vi "PLC_comm.vi"() -> ()   [LabVIEW 2017]
uses:
  <vilib>/DATA AHEAD/SP7/typedefs/PLC Type.ctl
  <vilib>/Utility/error.llb/DialogType.ctl
  <vilib>/addons/database/Connection.llb/DB Tools Open Connec (String).vi
  Global/Global 1.vi
  Global/DATA LOG.vi
  <vilib>/DATA AHEAD/SP7/functions/write/write Dint array.vi
  <vilib>/DATA AHEAD/SP7/functions/write/writeString.vi
  <vilib>/DATA AHEAD/SP7/functions/read/read Dint array.vi
  <vilib>/DATA AHEAD/SP7/functions/read/read real array.vi
  <vilib>/DATA AHEAD/SP7/functions/read/read String.vi
  <vilib>/addons/database/NI_Database_API.lvlib
  <vilib>/DATA AHEAD/SP7/SP7.lvlib
panel:
  out "IP1 7":string
  out "PLC 7":bool
  out "IP1 6":string
  out "PLC 6":bool
  out "IP1 5":string
  out "PLC 5":bool
  out "PLC 4":bool
  out "PLC 3":bool
  out "PLC 2":bool
  out "PLC 1":bool
  out "IP1 4":string
  out "IP1 3":string
  out "IP1 2":string
  out "IP1":string
  in  "stop":bool
  out "error out":errorcluster
  in  "error in (no error)":errorcluster
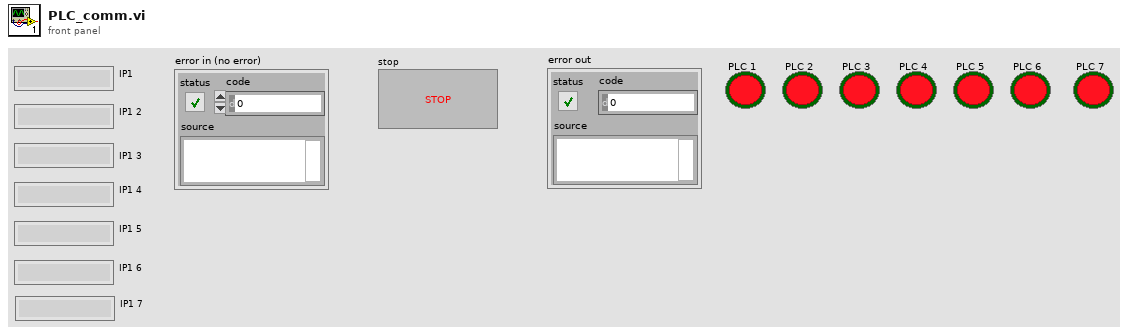
[diagram p1: front panel]
types:
  T1 = typedef "DialogType.ctl" = u16
  T2 = typedef "SP7.lvlib/PLC Type.ctl" = enum16{"S7 200", "S7 300/400", "S7 1200", "S7 1500", "LOGO!8"}
  T3 = typedef "NI_Database_API.lvlib/Conn ObjectReference.ctl" = refnum<k1>
  T4 = typedef "SP7.lvlib/S7 Connection.ctl" = cluster{"TCP Connection Ref":refnum<k5>, "IP address":string, "timeout ms":i32, "Connected?":bool, "PLC Type":T2, "Rack S7 400":u8, "Slot S7 400":u8, "PDU Size":u16, "connection semaphore":T5}
  T5 = typedef "Semaphore RefNum" = refnum<k1>
diagram:
  w2 = T1 0 items=["no dialog", "OK message", "continue or stop message", "OK message + warnings", "continue/stop + warnings"]  # type of dialog (OK msg:1)
  w4 = i32[] [0, 0, 0, 0, 0]  # I/P
  w5 = i32[] [0, 0]  # Input
  w7 = i32[] [0, 0]  # Input
  w8 = i32[] [0, 0]  # Input
  w10 = i32[] [0, 0]  # Input
  w6 = i32[] [0, 0, 0, 0, 0]  # I/P
  w9 = i32[] [0, 0, 0, 0, 0]  # I/P
  w11 = i32[] [0, 0, 0, 0, 0]  # I/P
  w12 = i32[] [0, 0, 0, 0, 0]  # I/P
  w13 = i32[] [0, 0]  # Input
  w14 = i32[] [0, 0]  # Input
  w15 = i32[] [0, 0, 0, 0, 0]  # I/P
  w16 = i32[] [0, 0, 0, 0, 0]  # I/P
  w17 = i32[] [0, 0]  # Input
  w18 = i32[] [0, 0]  # I/P
  w19 = i32[] [0, 0]  # Input
  # "OP 80"
  # "OP 70"
  # "OP 60"
  # "OP 50"
  # "OP 40"
  # "OP 30"
  # "OP 20"
  # "OP 10"
  n1 = call "path_db.vi"("error in"="error in (no error)") -> ("error out"=w174:errorcluster, "resulting string"=w179:string)  [unwired: 9 in]
  n2 = call-poly <vilib>:"DB Tools Open Connection.vi"("error in (no error)"=w174, "connection information"=w179) -> ("error out"=w178:errorcluster, "connection reference"=w177:T3)  [unwired: 6 in]
  n3 = call <vilib>:"DB Tools Select Data.vi"("error in (no error)"=w178, "columns"=string[] ["PLC_IP_1", "PLC_IP_2", "PLC_IP_3", "PLC_IP_4", "PLC_IP_5", "PLC_IP_6", "PLC_IP_7"], "table"="IP_SETTING", "connection reference"=w177) -> ("error out"=w176:errorcluster, "data"=w175:variant[][])  [unwired: 2 in, 1 out]
  n4 = call "PADMINI_varient_to_data.vi"("error in (no error)"=w176, "data"=w175) -> ("error out"=w26:errorcluster, "Array"=w170:string[][])  [unwired: 8 in]
  n5 = call "PADMINI_AUTO_CYCLE STATE.vi"("Enum"=enum16{"Read", "Write"}."Write", "error in (no error)"=w26, "Input"=w19) -> ("error out"=w156:errorcluster)  [unwired: 7 in, 1 out]
  n6 = Index Array(array=w170, index (row)=0) -> (element=w169:string[])  [unwired: 1 in]
  n7 = call "PADMINI_AUTO_BARCODE_STRING.vi"("Enum"=enum16{"Read", "Write"}."Write", "error in (no error)"=w156, "Input"=string[] ["", ""]) -> ("error out"=w153:errorcluster)  [unwired: 7 in, 1 out]
  n8 = call "PADMINI_AUTO_BARCODE_STATUS.vi"("Enum"=enum16{"Read", "Write"}."Write", "error in (no error)"=w153, "I/P"=w18) -> ("error out"=w151:errorcluster)  [unwired: 7 in, 1 out]
  n9 = call "PADMINI_AUTO_CYCLE VALUE 10.vi"("Enum"=enum16{"Read", "Write"}."Write", "error in (no error)"=w151, "Input"=dbl[] [0.0]) -> ("error out"=w145:errorcluster)  [unwired: 7 in, 1 out]
  n10 = call "PADMINI_AUTO_CYCLE STATE 20.vi"("Enum"=enum16{"Read", "Write"}."Write", "error in (no error)"=w145, "Input"=w5) -> ("error out"=w143:errorcluster)  [unwired: 7 in, 1 out]
  n11 = call "PADMINI_AUTO_CYCLE VALUE 20.vi"("Enum"=enum16{"Read", "Write"}."Write", "error in (no error)"=w143, "Input"=dbl[] [0.0, 0.0, 0.0, 0.0]) -> ("error out"=w139:errorcluster)  [unwired: 7 in, 1 out]
  n12 = call "PADMINI_AUTO_BARCODE_STRING2.vi"("Enum"=enum16{"Read", "Write"}."Write", "error in (no error)"=w139, "Input"=string[] ["", "", "", "", "", "", ""]) -> ("error out"=w137:errorcluster)  [unwired: 7 in, 1 out]
  n13 = call "PADMINI_AUTO_BARCODE_STATUS 20.vi"("Enum"=enum16{"Read", "Write"}."Write", "error in (no error)"=w137, "I/P"=w4) -> ("error out"=w131:errorcluster)  [unwired: 7 in, 1 out]
  n14 = call "PADMINI_AUTO_BARCODE_STATUS 30.vi"("Enum"=enum16{"Read", "Write"}."Write", "error in (no error)"=w131, "I/P"=w6) -> ("error out"=w128:errorcluster)  [unwired: 7 in, 1 out]
  n15 = call "PADMINI_AUTO_CYCLE STATE 30.vi"("Enum"=enum16{"Read", "Write"}."Write", "error in (no error)"=w128, "Input"=w7) -> ("error out"=w127:errorcluster)  [unwired: 7 in, 1 out]
  n16 = call "PADMINI_AUTO_CYCLE VALUE 30.vi"("Enum"=enum16{"Read", "Write"}."Write", "error in (no error)"=w127, "Input"=dbl[] [0.0, 0.0]) -> ("error out"=w124:errorcluster)  [unwired: 7 in, 1 out]
  n17 = call "PADMINI_AUTO_BARCODE_STRING 30.vi"("Enum"=enum16{"Read", "Write"}."Write", "error in (no error)"=w124, "Input"=string[] ["", "", ""]) -> ("error out"=w102:errorcluster)  [unwired: 7 in, 1 out]
  n18 = call "PADMINI_AUTO_BARCODE_STATUS 40.vi"("Enum"=enum16{"Read", "Write"}."Write", "error in (no error)"=w102, "I/P"=w9) -> ("error out"=w101:errorcluster)  [unwired: 7 in, 1 out]
  n19 = call "PADMINI_AUTO_CYCLE VALUE 40.vi"("Enum"=enum16{"Read", "Write"}."Write", "error in (no error)"=w101, "Input"=dbl[] [0.0, 0.0, 0.0, 0.0]) -> ("error out"=w100:errorcluster)  [unwired: 7 in, 1 out]
  n20 = call "PADMINI_AUTO_CYCLE STATE 40.vi"("Enum"=enum16{"Read", "Write"}."Write", "error in (no error)"=w100, "Input"=w8) -> ("error out"=w99:errorcluster)  [unwired: 7 in, 1 out]
  n21 = call "PADMINI_AUTO_BARCODE_STRING 40.vi"("Enum"=enum16{"Read", "Write"}."Write", "error in (no error)"=w99, "Input"=string[] ["", "", "", "", ""]) -> ("error out"=w81:errorcluster)  [unwired: 7 in, 1 out]
  n22 = call "PADMINI_AUTO_BARCODE_STATUS 50.vi"("Enum"=enum16{"Read", "Write"}."Write", "error in (no error)"=w81, "I/P"=w11) -> ("error out"=w83:errorcluster)  [unwired: 7 in, 1 out]
  n23 = call "PADMINI_AUTO_CYCLE STATE 50.vi"("Enum"=enum16{"Read", "Write"}."Write", "error in (no error)"=w83, "Input"=w10) -> ("error out"=w87:errorcluster)  [unwired: 7 in, 1 out]
  n24 = call "PADMINI_AUTO_CYCLE VALUE 50.vi"("Enum"=enum16{"Read", "Write"}."Write", "error in (no error)"=w87, "Input"=dbl[] [0.0, 0.0, 0.0]) -> ("error out"=w84:errorcluster)  [unwired: 7 in, 1 out]
  n25 = call "PADMINI_AUTO_BARCODE_STRING 50.vi"("Enum"=enum16{"Read", "Write"}."Write", "error in (no error)"=w84, "Input"=string[] ["", "", "", "", "", ""]) -> ("error out"=w59:errorcluster)  [unwired: 7 in, 1 out]
  n26 = call "PADMINI_AUTO_BARCODE_STATUS 60.vi"("Enum"=enum16{"Read", "Write"}."Write", "error in (no error)"=w59, "I/P"=w12) -> ("error out"=w63:errorcluster)  [unwired: 7 in, 1 out]
  n27 = call "PADMINI_AUTO_CYCLE STATE 60.vi"("Enum"=enum16{"Read", "Write"}."Write", "error in (no error)"=w63, "Input"=w13) -> ("error out"=w65:errorcluster)  [unwired: 7 in, 1 out]
  n28 = call "PADMINI_AUTO_CYCLE VALUE 60.vi"("Enum"=enum16{"Read", "Write"}."Write", "error in (no error)"=w65, "Input"=dbl[] [0.0, 0.0, 0.0, 0.0, 0.0]) -> ("error out"=w68:errorcluster)  [unwired: 7 in, 1 out]
  n29 = call "PADMINI_AUTO_BARCODE_STRING 60.vi"("Enum"=enum16{"Read", "Write"}."Write", "error in (no error)"=w68, "Input"=string[] ["", "", "", "", "", ""]) -> ("error out"=w35:errorcluster)  [unwired: 7 in, 1 out]
  n30 = call "PADMINI_AUTO_BARCODE_STATUS 70.vi"("Enum"=enum16{"Read", "Write"}."Write", "error in (no error)"=w35, "I/P"=w15) -> ("error out"=w38:errorcluster)  [unwired: 7 in, 1 out]
  n31 = call "PADMINI_AUTO_CYCLE STATE 70.vi"("Enum"=enum16{"Read", "Write"}."Read", "error in (no error)"=w38, "Input"=w14) -> ("error out"=w50:errorcluster)  [unwired: 7 in, 1 out]
  n32 = call "PADMINI_AUTO_CYCLE VALUE 70.vi"("Enum"=enum16{"Read", "Write"}."Write", "error in (no error)"=w50, "Input"=dbl[] [0.0, 0.0]) -> ("error out"=w47:errorcluster)  [unwired: 7 in, 1 out]
  n33 = call "PADMINI_AUTO_BARCODE_STRING 70.vi"("Enum"=enum16{"Read", "Write"}."Write", "error in (no error)"=w47, "Input"=string[] ["", ""]) -> ("error out"=w32:errorcluster)  [unwired: 7 in, 1 out]
  n34 = call "PADMINI_AUTO_BARCODE_STATUS 80.vi"("Enum"=enum16{"Read", "Write"}."Write", "error in (no error)"=w32, "I/P"=w16) -> ("error out"=w39:errorcluster)  [unwired: 7 in, 1 out]
  n35 = call "PADMINI_AUTO_CYCLE STATE 80.vi"("Enum"=enum16{"Read", "Write"}."Write", "error in (no error)"=w39, "Input"=w17) -> ("error out"=w43:errorcluster)  [unwired: 7 in, 1 out]
  n36 = call "PADMINI_AUTO_CYCLE VALUE 80.vi"("Enum"=enum16{"Read", "Write"}."Write", "error in (no error)"=w43, "Input"=sgl[] [0.0]) -> ("error out"=w46:errorcluster)  [unwired: 7 in, 1 out]
  n37 = call "PADMINI_AUTO_BARCODE_STRING 80.vi"("Enum"=enum16{"Read", "Write"}."Write", "error in (no error)"=w46, "Input"=string[] ["", "", ""]) -> ()  [unwired: 7 in, 2 out]
  n38 = Index Array(array=w169) -> (element #1=w118:string, element #2=w119:string, element #3=w113:string, element #4=w89:string, element #5=w71:string, element #6=w28:string, element #7=w27:string)  [unwired: 7 in]
  "IP1" <- w118
  "IP1 2" <- w119
  "IP1 3" <- w113
  "IP1 4" <- w89
  "IP1 5" <- w71
  "IP1 6" <- w28
  "IP1 7" <- w27
  n39 = call <vilib>:"connect.vi"("PLC Type"=PLC_Type."S7 1200" ("PLC Type 2"), "error in (no error)"=w26, "timeout [ms]"=1000 ("timeout [ms] 2"), "IP address"=w27) -> ("error out"=w29:errorcluster, "S7 Connection out"=w1:T4)  [unwired: 6 in]
  n40 = call <vilib>:"connect.vi"("PLC Type"=PLC_Type."S7 1200" ("PLC Type 2"), "error in (no error)"=w26, "timeout [ms]"=1000 ("timeout [ms] 2"), "IP address"=w71) -> ("error out"=w76:errorcluster, "S7 Connection out"=w75:T4)  [unwired: 6 in]
  n41 = call <vilib>:"connect.vi"("PLC Type"=PLC_Type."S7 1200" ("PLC Type 2"), "error in (no error)"=w26, "timeout [ms]"=1000 ("timeout [ms] 2"), "IP address"=w28) -> ("error out"=w56:errorcluster, "S7 Connection out"=w55:T4)  [unwired: 6 in]
  n42 = call <vilib>:"connect.vi"("PLC Type"=PLC_Type."S7 1200" ("PLC Type 2"), "error in (no error)"=w26, "timeout [ms]"=1000 ("timeout [ms] 2"), "IP address"=w89) -> ("error out"=w92:errorcluster, "S7 Connection out"=w93:T4)  [unwired: 6 in]
  n43 = call <vilib>:"connect.vi"("PLC Type"=PLC_Type."S7 1200" ("PLC Type 2"), "error in (no error)"=w26, "timeout [ms]"=1000 ("timeout [ms] 2"), "IP address"=w119) -> ("error out"=w134:errorcluster, "S7 Connection out"=w133:T4)  [unwired: 6 in]
  n44 = call <vilib>:"connect.vi"("PLC Type"=PLC_Type."S7 1200" ("PLC Type 2"), "error in (no error)"=w26, "timeout [ms]"=1000 ("timeout [ms] 2"), "IP address"=w113) -> ("error out"=w115:errorcluster, "S7 Connection out"=w114:T4)  [unwired: 6 in]
  n45 = call <vilib>:"connect.vi"("PLC Type"=PLC_Type."S7 1200" ("PLC Type 2"), "error in (no error)"=w26, "timeout [ms]"=1000, "IP address"=w118) -> ("error out"=w160:errorcluster, "S7 Connection out"=w159:T4)  [unwired: 6 in]
  n46 = while {
    shift-right: [w182] -> w23
    shift-left: w1 -> [w192]
    shift-right: [w190] -> w24
    shift-left: w29 -> [w191]
    tunnel: w27 -> [w181]
    stop <- w184 stop-if-true
    # "OP 90 - 100 - 110"
    n47 = flat-sequence {
      tunnel: [w268] -> w188
      tunnel: [w269] -> w183
      tunnel: w191 -> [w307]
      tunnel: w192 -> [w306]
      tunnel: w181 -> [w288]
      tunnel: [w288] -> w180
      tunnel: [w375] -> w190
      tunnel: [w374] -> w182
      tunnel: w188 -> [w377]
      tunnel: w183 -> [w376]
      tunnel: w180 -> [w373]
      frame #0 {
        w209 = u16 75 ("Data Block #")
        w234 = u16 72 ("Data Block #")
        w260 = u16 70 ("Data Block #")
        w218 = u16 71 ("Data Block #")
        w248 = u16 69 ("Data Block #")
        # "OP100 OK\nOP 100 NG"
        # "AUTO WRITE"
        n48 = global read "DATA LOG.vi" "OP 90 Outputs"() -> (w305:bool)
        n49 = case shown="True" w305 {
          tunnel: w306 -> [w358 w371]
          tunnel: [w359 w360] -> w265
          tunnel: [w358 w361] -> w266
          tunnel: w307 -> [w359 w368]
          frame False {
          }
          frame True {
            w372 = u16 70  # Data Block #
            n50 = call "PADMINI_AUTO_BARCODE_STATUS 90.vi"("Enum"=enum16{"Read", "Write"}."Read", "error in (no error)"=w368) -> ("error out"=w367:errorcluster, "O/P"=w369:i32[])  [unwired: 8 in]
            n51 = global write "DATA LOG.vi" "OP 90 Outputs"(FALSE) -> ()
            n52 = call-poly <vilib>:"write DB.vi"("DINT input array"=w369, "error in (no error)"=w367, "Data Block #"=w372, "S7 Connection in"=w371) -> ("error out"=w363:errorcluster, "S7 Connection out"=w362:T4)  [unwired: 4 in, 2 out]
            n53 = call-poly <vilib>:"write DB.vi"("DINT input array"=i32[] [0] ("Data Byte"), "error in (no error)"=w363, "Data Block #"=u16 69, "S7 Connection in"=w362) -> ("error out"=w360:errorcluster, "S7 Connection out"=w361:T4)  [unwired: 4 in, 2 out]
          }
        }
        n54 = global read "DATA LOG.vi" "OP 90 reset"() -> (w264:bool)
        n55 = case shown="True" w264 {
          tunnel: w265 -> [w333 w342]
          tunnel: [w333 w341] -> w253
          tunnel: w266 -> [w334 w340]
          tunnel: [w334 w339] -> w254
          frame False {
          }
          frame True {
            n56 = global write "DATA LOG.vi" "OP 90 reset"(FALSE) -> ()
            n57 = call-poly <vilib>:"write DB.vi"("Item offset [byte]"=u16 4 ("Data Block #"), "DINT input array"=i32[] [0], "error in (no error)"=w342, "Data Block #"=u16 69, "S7 Connection in"=w340) -> ("error out"=w341:errorcluster, "S7 Connection out"=w339:T4)  [unwired: 3 in, 2 out]
          }
        }
        n58 = global read "DATA LOG.vi" "Auto Cycle On"() -> (w200:bool)
        n59 = Boolean To (0,1)(Boolean=w200) -> (0, 1=w199:i16)
        n60 = Build Array(w199) -> (w198:i16[])
        n61 = global read "Global 1.vi" "Filtered BARCODE selected"() -> (w263:string[])
        n62 = call-poly <vilib>:"write DB.vi"("Item offset [byte]"=u32 20, "DINT input array"=w198, "error in (no error)"=w253, "Data Block #"=w260, "S7 Connection in"=w254) -> ("error out"=w258:errorcluster, "S7 Connection out"=w257:T4)  [unwired: 3 in, 2 out]
        n63 = call-poly <vilib>:"write DB.vi"("Item offset [byte]"=u32 24, "Input STRINGS"=w263, "error in (no error)"=w258, "String length reserved in DB (default=254)"=u16 15, "Data Block #"=w260, "S7 Connection in"=w257) -> ("error out"=w255:errorcluster, "S7 Connection out"=w256:T4)  [unwired: 2 in, 2 out]
        n64 = call-poly <vilib>:"read DB.vi"("error in (no error)"=w255, "items #"=u16 2 ("Items # [byte]"), "Data Block #"=w248, "S7 Connection in"=w256) -> ("error out"=w303:errorcluster, "DINT result array"=w301:i32[], "S7 Connection out"=w298:T4)  [unwired: 5 in]
        n65 = call "PADMINI_AUTO_CYCLE STATE 90.vi"("Enum"=enum16{"Read", "Write"}."Write", "error in (no error)"=w303, "Input"=w301) -> ("error out"=w299:errorcluster)  [unwired: 7 in, 1 out]
        n66 = call-poly <vilib>:"read DB.vi"("Item offset [byte]"=u32 8, "error in (no error)"=w299, "items #"=u16 2 ("Items # [byte]"), "Data Block #"=w248, "S7 Connection in"=w298) -> ("error out"=w291:errorcluster, "REAL result array"=w289:sgl[], "S7 Connection out"=w297:T4)  [unwired: 4 in]
        n67 = call "PADMINI_AUTO_CYCLE VALUE 90.vi"("Enum"=enum16{"Read", "Write"}."Write", "error in (no error)"=w291, "Input"=w289) -> ("error out"=w290:errorcluster)  [unwired: 7 in, 1 out]
        n68 = call-poly <vilib>:"read DB.vi"("Item offset [byte]"=u32 16, "String length reserved in DB (default=254)"=u16 50, "error in (no error)"=w290, "items #"=u16 1 ("Items # [byte]"), "Data Block #"=w248, "S7 Connection in"=w297) -> ("error out"=w252:errorcluster, "STRING result Array"=w243:string[], "S7 Connection out"=w251:T4)  [unwired: 2 in, 1 out]
        n69 = call-poly <vilib>:"read DB.vi"("Item offset [byte]"=u32 68, "String length reserved in DB (default=254)"=u16 10, "error in (no error)"=w252, "items #"=u16 3 ("Items # [byte]"), "Data Block #"=w248, "S7 Connection in"=w251) -> ("error out"=w250:errorcluster, "STRING result Array"=w242:string[], "S7 Connection out"=w249:T4)  [unwired: 2 in, 1 out]
        n70 = Build Array (concatenate)(w243, w242) -> (w241:string[])
        n71 = call "PADMINI_AUTO_BARCODE_STRING 90.vi"("Enum"=enum16{"Read", "Write"}."Write", "error in (no error)"=w250, "Input"=w241) -> ("error out"=w270:errorcluster)  [unwired: 7 in, 1 out]
        n72 = global read "DATA LOG.vi" "OP 100 Outputs"() -> (w271:bool)
        n73 = case shown="True" w271 {
          tunnel: w249 -> [w343 w356]
          tunnel: [w344 w347] -> w239
          tunnel: [w343 w348] -> w240
          tunnel: w270 -> [w344 w353]
          frame False {
          }
          frame True {
            w357 = u16 72  # Data Block #
            n74 = call "PADMINI_AUTO_BARCODE_STATUS 100.vi"("Enum"=enum16{"Read", "Write"}."Read", "error in (no error)"=w353) -> ("error out"=w352:errorcluster, "O/P"=w354:i32[])  [unwired: 8 in]
            n75 = global write "DATA LOG.vi" "OP 100 Outputs"(FALSE) -> ()
            n76 = call-poly <vilib>:"write DB.vi"("DINT input array"=w354, "error in (no error)"=w352, "Data Block #"=w357, "S7 Connection in"=w356) -> ("error out"=w346:errorcluster, "S7 Connection out"=w345:T4)  [unwired: 4 in, 2 out]
            n77 = call-poly <vilib>:"write DB.vi"("DINT input array"=i32[] [0] ("Data Byte"), "error in (no error)"=w346, "Data Block #"=u16 71, "S7 Connection in"=w345) -> ("error out"=w347:errorcluster, "S7 Connection out"=w348:T4)  [unwired: 4 in, 2 out]
          }
        }
        n78 = global read "DATA LOG.vi" "OP 100 reset"() -> (w238:bool)
        n79 = case shown="True" w238 {
          tunnel: w239 -> [w323 w332]
          tunnel: [w323 w331] -> w230
          tunnel: w240 -> [w324 w330]
          tunnel: [w324 w329] -> w229
          frame False {
          }
          frame True {
            n80 = global write "DATA LOG.vi" "OP 100 reset"(FALSE) -> ()
            n81 = call-poly <vilib>:"write DB.vi"("Item offset [byte]"=u16 4 ("Data Block #"), "DINT input array"=i32[] [0], "error in (no error)"=w332, "Data Block #"=u16 71, "S7 Connection in"=w330) -> ("error out"=w331:errorcluster, "S7 Connection out"=w329:T4)  [unwired: 3 in, 2 out]
          }
        }
        n82 = global read "DATA LOG.vi" "Auto Cycle On"() -> (w197:bool)
        n83 = Boolean To (0,1)(Boolean=w197) -> (0, 1=w196:i16)
        n84 = Build Array(w196) -> (w195:i16[])
        n85 = global read "Global 1.vi" "Filtered BARCODE selected"() -> (w231:string[])
        n86 = call-poly <vilib>:"write DB.vi"("Item offset [byte]"=u32 20, "DINT input array"=w195, "error in (no error)"=w230, "Data Block #"=w234, "S7 Connection in"=w229) -> ("error out"=w236:errorcluster, "S7 Connection out"=w237:T4)  [unwired: 3 in, 2 out]
        n87 = call-poly <vilib>:"write DB.vi"("Item offset [byte]"=u32 24, "Input STRINGS"=w231, "error in (no error)"=w236, "String length reserved in DB (default=254)"=u16 15, "Data Block #"=w234, "S7 Connection in"=w237) -> ("error out"=w227:errorcluster, "S7 Connection out"=w228:T4)  [unwired: 2 in, 2 out]
        n88 = call-poly <vilib>:"read DB.vi"("error in (no error)"=w227, "items #"=u16 2 ("Items # [byte]"), "Data Block #"=w218, "S7 Connection in"=w228) -> ("error out"=w273:errorcluster, "DINT result array"=w275:i32[], "S7 Connection out"=w278:T4)  [unwired: 5 in]
        n89 = call "PADMINI_AUTO_CYCLE STATE 100.vi"("Enum"=enum16{"Read", "Write"}."Write", "error in (no error)"=w273, "Input"=w275) -> ("error out"=w277:errorcluster)  [unwired: 7 in, 1 out]
        n90 = call-poly <vilib>:"read DB.vi"("Item offset [byte]"=u32 8, "error in (no error)"=w277, "items #"=u16 11 ("Items # [byte]"), "Data Block #"=w218, "S7 Connection in"=w278) -> ("error out"=w285:errorcluster, "REAL result array"=w287:sgl[], "S7 Connection out"=w279:T4)  [unwired: 4 in]
        n91 = call "PADMINI_AUTO_CYCLE VALUE 100.vi"("Enum"=enum16{"Read", "Write"}."Write", "error in (no error)"=w285, "Input"=w287) -> ("error out"=w286:errorcluster)  [unwired: 7 in, 1 out]
        n92 = call-poly <vilib>:"read DB.vi"("Item offset [byte]"=u32 52, "String length reserved in DB (default=254)"=u16 50, "error in (no error)"=w286, "items #"=u16 1 ("Items # [byte]"), "Data Block #"=w218, "S7 Connection in"=w279) -> ("error out"=w224:errorcluster, "STRING result Array"=w221:string[], "S7 Connection out"=w223:T4)  [unwired: 2 in, 1 out]
        n93 = call-poly <vilib>:"read DB.vi"("Item offset [byte]"=u32 104, "String length reserved in DB (default=254)"=u16 10, "error in (no error)"=w224, "items #"=u16 2 ("Items # [byte]"), "Data Block #"=w218, "S7 Connection in"=w223) -> ("error out"=w225:errorcluster, "STRING result Array"=w219:string[], "S7 Connection out"=w222:T4)  [unwired: 2 in, 1 out]
        n94 = Build Array (concatenate)(w221, w219) -> (w220:string[])
        n95 = call "PADMINI_AUTO_BARCODE_STRING 100.vi"("Enum"=enum16{"Read", "Write"}."Write", "error in (no error)"=w225, "Input"=w220) -> ("error out"=w267:errorcluster)  [unwired: 7 in, 1 out]
        n96 = global read "DATA LOG.vi" "OP 110 Outputs"() -> (w215:bool)
        n97 = case shown="True" w215 {
          tunnel: [w308 w313] -> w201
          tunnel: [w309 w314] -> w202
          tunnel: w267 -> [w308 w318]
          tunnel: w222 -> [w309 w317]
          frame False {
          }
          frame True {
            w310 = i32[] [0]  # DINT input array
            w311 = u16 75  # Data Block #
            n98 = call "PADMINI_AUTO_BARCODE_STATUS 110.vi"("Enum"=enum16{"Read", "Write"}."Read", "error in (no error)"=w318) -> ("error out"=w320:errorcluster, "O/P"=w321:i32[])  [unwired: 8 in]
            n99 = call-poly <vilib>:"write DB.vi"("Item offset [byte]"=u32 4, "DINT input array"=w321, "error in (no error)"=w320, "Data Block #"=w311, "S7 Connection in"=w317) -> ("error out"=w312:errorcluster, "S7 Connection out"=w315:T4)  [unwired: 3 in, 2 out]
            n100 = global write "DATA LOG.vi" "OP 110 Outputs"(FALSE) -> ()
            n101 = call-poly <vilib>:"write DB.vi"("DINT input array"=w310, "error in (no error)"=w312, "Data Block #"=w311, "S7 Connection in"=w315) -> ("error out"=w313:errorcluster, "S7 Connection out"=w314:T4)  [unwired: 4 in, 2 out]
          }
        }
        n102 = call-poly <vilib>:"read DB.vi"("error in (no error)"=w201, "items #"=u16 1 ("Items # [byte]"), "Data Block #"=w209, "S7 Connection in"=w202) -> ("error out"=w213:errorcluster, "DINT result array"=w211:i32[], "S7 Connection out"=w210:T4)  [unwired: 5 in]
        n103 = call "PADMINI_AUTO_CYCLE STATE 110.vi"("Enum"=enum16{"Read", "Write"}."Write", "error in (no error)"=w213, "Input"=w211) -> ("error out"=w203:errorcluster)  [unwired: 7 in, 1 out]
        n104 = call-poly <vilib>:"read DB.vi"("Item offset [byte]"=u32 12, "String length reserved in DB (default=254)"=u16 50, "error in (no error)"=w203, "items #"=u16 1 ("Items # [byte]"), "Data Block #"=w209, "S7 Connection in"=w210) -> ("error out"=w205:errorcluster, "STRING result Array"=w206:string[], "S7 Connection out"=w268:T4)  [unwired: 2 in, 1 out]
        n105 = call "PADMINI_AUTO_BARCODE_STRING 110.vi"("Enum"=enum16{"Read", "Write"}."Write", "error in (no error)"=w205, "Input"=w206) -> ("error out"=w269:errorcluster)  [unwired: 7 in, 1 out]
      }
      frame #1 {
        # "RECONNECT"
        n106 = case shown="Error" w376 {
          selector: w376 -> [w381 w389]
          tunnel: [w380 w386] -> w374
          tunnel: [w381 w387] -> w375
          tunnel: w377 -> [w380 w383]
          tunnel: w373 -> [_ w382]
          frame No Error {
          }
          frame Error {
            n107 = call <vilib>:"Clear Errors.vi"("error in (no error)"=w389) -> ("error out"=w390:errorcluster)  [unwired: 5 in, 1 out]
            n108 = call <vilib>:"disconnect.vi"("error in (no error)"=w390, "S7 Connection in"=w383) -> ("error out"=w388:errorcluster)  [unwired: 8 in, 1 out]
            n109 = call <vilib>:"Clear Errors.vi"("error in (no error)"=w388) -> ("error out"=w385:errorcluster)  [unwired: 5 in, 1 out]
            n110 = call <vilib>:"connect.vi"("PLC Type"=PLC_Type."S7 1200" ("PLC Type 2"), "error in (no error)"=w385, "IP address"=w382) -> ("error out"=w387:errorcluster, "S7 Connection out"=w386:T4)  [unwired: 7 in]
          }
        }
        n111 = Unbundle By Name(w376) -> ("status"=w379:bool)
        n112 = Not(x=w379) -> (.not. x?=w378:bool)
        "PLC 7" <- w378
        n113 = global write "Global 1.vi" "PLC 7"(w378) -> ()
      }
    }
    n114 = call "PADMINI_STOP_ALL.vi"("Enum"=enum16{"Read", "Write"}."Read") -> ("Boolean 2"=w186:bool)  [unwired: 9 in, 1 out]
    n115 = local read "stop"() -> (w185:bool)
    n116 = Or(x=w185, y=w186) -> (x .or. y?=w184:bool)
    n117 = Wait (ms)(milliseconds to wait=u32 50) -> ()  [unwired: 1 out]
  }
  n118 = while {
    shift-right: [w393] -> w121
    shift-left: w133 -> [w403]
    shift-right: [w401] -> w120
    shift-left: w134 -> [w402]
    tunnel: w119 -> [w392]
    stop <- w395 stop-if-true
    # "OP 30"
    n119 = flat-sequence {
      tunnel: [w406] -> w399
      tunnel: [w408] -> w394
      tunnel: w402 -> [w410]
      tunnel: w403 -> [w409]
      tunnel: w392 -> [w407]
      tunnel: [w407] -> w391
      tunnel: [w413] -> w401
      tunnel: [w412] -> w393
      tunnel: w399 -> [w415]
      tunnel: w394 -> [w414]
      tunnel: w391 -> [w411]
      frame #0 {
        # "AUTO WRITE"
        n120 = call "PLC_OP30_Write.vi"("error in (no error)"=w410, "S7 Connection in"=w409) -> ("error out"=w404:errorcluster, "S7 Connection out"=w405:T4)  [unwired: 8 in]
        n121 = call "PLC_OP30_Read.vi"("error in (no error)"=w404, "S7 Connection in"=w405) -> ("error out"=w408:errorcluster, "S7 Connection out 2"=w406:T4)  [unwired: 8 in]
      }
      frame #1 {
        # "RECONNECT"
        n122 = case shown="Error" w414 {
          selector: w414 -> [w419 w427]
          tunnel: [w418 w424] -> w412
          tunnel: [w419 w425] -> w413
          tunnel: w415 -> [w418 w421]
          tunnel: w411 -> [_ w420]
          frame No Error {
          }
          frame Error {
            n123 = call <vilib>:"Clear Errors.vi"("error in (no error)"=w427) -> ("error out"=w428:errorcluster)  [unwired: 5 in, 1 out]
            n124 = call <vilib>:"disconnect.vi"("error in (no error)"=w428, "S7 Connection in"=w421) -> ("error out"=w426:errorcluster)  [unwired: 8 in, 1 out]
            n125 = call <vilib>:"Clear Errors.vi"("error in (no error)"=w426) -> ("error out"=w423:errorcluster)  [unwired: 5 in, 1 out]
            n126 = call <vilib>:"connect.vi"("PLC Type"=PLC_Type."S7 1200" ("PLC Type 2"), "error in (no error)"=w423, "IP address"=w420) -> ("error out"=w425:errorcluster, "S7 Connection out"=w424:T4)  [unwired: 7 in]
          }
        }
        n127 = Unbundle By Name(w414) -> ("status"=w417:bool)
        n128 = Not(x=w417) -> (.not. x?=w416:bool)
        "PLC 2" <- w416
        n129 = global write "Global 1.vi" "PLC 2"(w416) -> ()
      }
    }
    n130 = call "PADMINI_STOP_ALL.vi"("Enum"=enum16{"Read", "Write"}."Read") -> ("Boolean 2"=w397:bool)  [unwired: 9 in, 1 out]
    n131 = Wait (ms)(milliseconds to wait=u32 50) -> ()  [unwired: 1 out]
    n132 = local read "stop"() -> (w396:bool)
    n133 = Or(x=w396, y=w397) -> (x .or. y?=w395:bool)
  }
  n134 = while {
    shift-right: [w431] -> w148
    shift-left: w159 -> [w441]
    shift-right: [w439] -> w163
    shift-left: w160 -> [w440]
    tunnel: w118 -> [w429]
    stop <- w434 stop-if-true
    # "OP 10 AND 20"
    n135 = flat-sequence {
      tunnel: [w444] -> w433
      tunnel: [w450] -> w432
      tunnel: w440 -> [w451]
      tunnel: w441 -> [w452]
      tunnel: [w449] -> w430
      tunnel: w429 -> [w449]
      tunnel: [w456] -> w439
      tunnel: [w455] -> w431
      tunnel: w433 -> [w457]
      tunnel: w432 -> [w453]
      tunnel: w430 -> [w454]
      frame #0 {
        # "NEW CHANGES"
        n136 = call "PLC_OP10_Write.vi"("error in (no error)"=w451, "S7 Connection in"=w452) -> ("error out"=w447:errorcluster, "S7 Connection out"=w448:T4)  [unwired: 8 in]
        n137 = call "PLC_OP10_Read.vi"("error in (no error)"=w447, "S7 Connection in"=w448) -> ("error out"=w446:errorcluster, "S7 Connection out"=w445:T4)  [unwired: 8 in]
        n138 = call "PLC_OP20_Write.vi"("error in (no error)"=w446, "S7 Connection in"=w445) -> ("error out"=w442:errorcluster, "S7 Connection out"=w443:T4)  [unwired: 8 in]
        n139 = call "PLC_OP20_Read.vi"("error in (no error)"=w442, "S7 Connection in"=w443) -> ("error out"=w450:errorcluster, "S7 Connection out 2"=w444:T4)  [unwired: 8 in]
      }
      frame #1 {
        # "RECONNECT"
        n140 = Unbundle By Name(w453) -> ("status"=w459:bool)
        n141 = case shown="Error" w453 {
          selector: w453 -> [w461 w470]
          tunnel: [w460 w467] -> w455
          tunnel: [w461 w468] -> w456
          tunnel: w457 -> [w460 w464]
          tunnel: w454 -> [_ w463]
          frame No Error {
          }
          frame Error {
            w462 = 1000  # timeout [ms]
            n142 = call <vilib>:"Clear Errors.vi"("error in (no error)"=w470) -> ("error out"=w471:errorcluster)  [unwired: 5 in, 1 out]
            n143 = call <vilib>:"disconnect.vi"("error in (no error)"=w471, "S7 Connection in"=w464) -> ("error out"=w469:errorcluster)  [unwired: 8 in, 1 out]
            n144 = call <vilib>:"Clear Errors.vi"("error in (no error)"=w469) -> ("error out"=w466:errorcluster)  [unwired: 5 in, 1 out]
            n145 = call <vilib>:"connect.vi"("PLC Type"=PLC_Type."S7 1200" ("PLC Type 2"), "error in (no error)"=w466, "timeout [ms]"=w462, "IP address"=w463) -> ("error out"=w468:errorcluster, "S7 Connection out"=w467:T4)  [unwired: 6 in]
          }
        }
        n146 = Not(x=w459) -> (.not. x?=w458:bool)
        "PLC 1" <- w458
        n147 = global write "Global 1.vi" "PLC 1"(w458) -> ()
      }
    }
    n148 = call "PADMINI_STOP_ALL.vi"("Enum"=enum16{"Read", "Write"}."Read") -> ("Boolean 2"=w436:bool)  [unwired: 9 in, 1 out]
    n149 = Or(x="stop", y=w436) -> (x .or. y?=w434:bool)
    n150 = Wait (ms)(milliseconds to wait=u32 50) -> ()  [unwired: 1 out]
  }
  n151 = while {
    shift-right: [w474] -> w96
    shift-left: w93 -> [w484]
    shift-right: [w482] -> w95
    shift-left: w92 -> [w483]
    tunnel: w89 -> [w473]
    stop <- w476 stop-if-true
    # "OP 50"
    n152 = flat-sequence {
      tunnel: [w505] -> w480
      tunnel: [w515] -> w475
      tunnel: w483 -> [w534]
      tunnel: w484 -> [w533]
      tunnel: w473 -> [w514]
      tunnel: [w514] -> w472
      tunnel: [w562] -> w482
      tunnel: [w561] -> w474
      tunnel: w480 -> [w564]
      tunnel: w475 -> [w563]
      tunnel: w472 -> [w560]
      frame #0 {
        w496 = u16 57 ("Data Block #")
        w504 = u16 56 ("Data Block #")
        # "AUTO WRITE"
        n153 = global read "DATA LOG.vi" "OP 50 Outputs"() -> (w532:bool)
        n154 = case shown="True" w532 {
          tunnel: w533 -> [w545 w558]
          tunnel: [w546 w547] -> w513
          tunnel: [w545 w550] -> w512
          tunnel: w534 -> [w546 w555]
          frame False {
          }
          frame True {
            w559 = u16 57  # Data Block #
            n155 = call "PADMINI_AUTO_BARCODE_STATUS 50.vi"("Enum"=enum16{"Read", "Write"}."Read", "error in (no error)"=w555) -> ("error out"=w554:errorcluster, "O/P"=w556:i32[])  [unwired: 8 in]
            n156 = global write "DATA LOG.vi" "OP 50 Outputs"(FALSE) -> ()
            n157 = call-poly <vilib>:"write DB.vi"("DINT input array"=w556, "error in (no error)"=w554, "Data Block #"=w559, "S7 Connection in"=w558) -> ("error out"=w548:errorcluster, "S7 Connection out"=w549:T4)  [unwired: 4 in, 2 out]
            n158 = call-poly <vilib>:"write DB.vi"("DINT input array"=i32[] [0] ("Data Byte"), "error in (no error)"=w548, "Data Block #"=u16 56, "S7 Connection in"=w549) -> ("error out"=w547:errorcluster, "S7 Connection out"=w550:T4)  [unwired: 4 in, 2 out]
          }
        }
        n159 = global read "DATA LOG.vi" "OP 50 reset"() -> (w511:bool)
        n160 = global read "DATA LOG.vi" "Auto Cycle On"() -> (w487:bool)
        n161 = case shown="True" w511 {
          tunnel: w513 -> [w535 w544]
          tunnel: [w535 w543] -> w489
          tunnel: w512 -> [w536 w542]
          tunnel: [w536 w541] -> w492
          frame False {
          }
          frame True {
            n162 = global write "DATA LOG.vi" "OP 50 reset"(FALSE) -> ()
            n163 = call-poly <vilib>:"write DB.vi"("Item offset [byte]"=u16 4 ("Data Block #"), "DINT input array"=i32[] [0], "error in (no error)"=w544, "Data Block #"=u16 56, "S7 Connection in"=w542) -> ("error out"=w543:errorcluster, "S7 Connection out"=w541:T4)  [unwired: 3 in, 2 out]
          }
        }
        n164 = Boolean To (0,1)(Boolean=w487) -> (0, 1=w486:i16)
        n165 = Build Array(w486) -> (w485:i16[])
        n166 = global read "Global 1.vi" "Filtered BARCODE selected"() -> (w493:string[])
        n167 = call-poly <vilib>:"write DB.vi"("Item offset [byte]"=u32 20, "DINT input array"=w485, "error in (no error)"=w489, "Data Block #"=w496, "S7 Connection in"=w492) -> ("error out"=w498:errorcluster, "S7 Connection out"=w499:T4)  [unwired: 3 in, 2 out]
        n168 = call-poly <vilib>:"write DB.vi"("Item offset [byte]"=u32 24, "Input STRINGS"=w493, "error in (no error)"=w498, "String length reserved in DB (default=254)"=u16 15, "Data Block #"=w496, "S7 Connection in"=w499) -> ("error out"=w490:errorcluster, "S7 Connection out"=w491:T4)  [unwired: 2 in, 2 out]
        n169 = call-poly <vilib>:"read DB.vi"("error in (no error)"=w490, "items #"=u16 2 ("Items # [byte]"), "Data Block #"=w504, "S7 Connection in"=w491) -> ("error out"=w530:errorcluster, "DINT result array"=w528:i32[], "S7 Connection out"=w525:T4)  [unwired: 5 in]
        n170 = call "PADMINI_AUTO_CYCLE STATE 50.vi"("Enum"=enum16{"Read", "Write"}."Write", "error in (no error)"=w530, "Input"=w528) -> ("error out"=w526:errorcluster)  [unwired: 7 in, 1 out]
        n171 = call-poly <vilib>:"read DB.vi"("Item offset [byte]"=u32 8, "error in (no error)"=w526, "items #"=u16 3 ("Items # [byte]"), "Data Block #"=w504, "S7 Connection in"=w525) -> ("error out"=w518:errorcluster, "REAL result array"=w516:sgl[], "S7 Connection out"=w524:T4)  [unwired: 4 in]
        n172 = call "PADMINI_AUTO_CYCLE VALUE 50.vi"("Enum"=enum16{"Read", "Write"}."Write", "error in (no error)"=w518, "Input"=w516) -> ("error out"=w517:errorcluster)  [unwired: 7 in, 1 out]
        n173 = call-poly <vilib>:"read DB.vi"("Item offset [byte]"=u32 20, "String length reserved in DB (default=254)"=u16 50, "error in (no error)"=w517, "items #"=u16 1 ("Items # [byte]"), "Data Block #"=w504, "S7 Connection in"=w524) -> ("error out"=w507:errorcluster, "STRING result Array"=w503:string[], "S7 Connection out"=w506:T4)  [unwired: 2 in, 1 out]
        n174 = call-poly <vilib>:"read DB.vi"("Item offset [byte]"=u32 72, "String length reserved in DB (default=254)"=u16 10, "error in (no error)"=w507, "items #"=u16 5 ("Items # [byte]"), "Data Block #"=w504, "S7 Connection in"=w506) -> ("error out"=w508:errorcluster, "STRING result Array"=w502:string[], "S7 Connection out"=w505:T4)  [unwired: 2 in, 1 out]
        n175 = Build Array (concatenate)(w503, w502) -> (w501:string[])
        n176 = call "PADMINI_AUTO_BARCODE_STRING 50.vi"("Enum"=enum16{"Read", "Write"}."Write", "error in (no error)"=w508, "Input"=w501) -> ("error out"=w515:errorcluster)  [unwired: 7 in, 1 out]
      }
      frame #1 {
        # "RECONNECT"
        n177 = case shown="Error" w563 {
          selector: w563 -> [w568 w576]
          tunnel: [w567 w573] -> w561
          tunnel: [w568 w574] -> w562
          tunnel: w564 -> [w567 w570]
          tunnel: w560 -> [_ w569]
          frame No Error {
          }
          frame Error {
            n178 = call <vilib>:"Clear Errors.vi"("error in (no error)"=w576) -> ("error out"=w577:errorcluster)  [unwired: 5 in, 1 out]
            n179 = call <vilib>:"disconnect.vi"("error in (no error)"=w577, "S7 Connection in"=w570) -> ("error out"=w575:errorcluster)  [unwired: 8 in, 1 out]
            n180 = call <vilib>:"Clear Errors.vi"("error in (no error)"=w575) -> ("error out"=w572:errorcluster)  [unwired: 5 in, 1 out]
            n181 = call <vilib>:"connect.vi"("PLC Type"=PLC_Type."S7 1200" ("PLC Type 2"), "error in (no error)"=w572, "IP address"=w569) -> ("error out"=w574:errorcluster, "S7 Connection out"=w573:T4)  [unwired: 7 in]
          }
        }
        n182 = Unbundle By Name(w563) -> ("status"=w566:bool)
        n183 = Not(x=w566) -> (.not. x?=w565:bool)
        "PLC 4" <- w565
        n184 = global write "Global 1.vi" "PLC 4"(w565) -> ()
      }
    }
    n185 = call "PADMINI_STOP_ALL.vi"("Enum"=enum16{"Read", "Write"}."Read") -> ("Boolean 2"=w478:bool)  [unwired: 9 in, 1 out]
    n186 = local read "stop"() -> (w477:bool)
    n187 = Or(x=w477, y=w478) -> (x .or. y?=w476:bool)
    n188 = Wait (ms)(milliseconds to wait=u32 50) -> ()  [unwired: 1 out]
  }
  n189 = while {
    shift-right: [w580] -> w52
    shift-left: w55 -> [w590]
    shift-right: [w588] -> w53
    shift-left: w56 -> [w589]
    tunnel: w28 -> [w579]
    stop <- w582 stop-if-true
    # "OP 70 - 80"
    n190 = flat-sequence {
      tunnel: [w601] -> w586
      tunnel: [w649] -> w581
      tunnel: w589 -> [w687]
      tunnel: w590 -> [w686]
      tunnel: w579 -> [w668]
      tunnel: [w668] -> w578
      tunnel: [w740] -> w588
      tunnel: [w739] -> w580
      tunnel: w586 -> [w742]
      tunnel: w581 -> [w741]
      tunnel: w578 -> [w738]
      frame #0 {
        w617 = u16 83 ("Data Block #")
        w642 = u16 81 ("Data Block #")
        w600 = u16 82 ("Data Block #")
        w623 = u16 80 ("Data Block #")
        # "AUTO WRITE"
        n191 = global read "DATA LOG.vi" "OP 70 Outputs"() -> (w685:bool)
        n192 = case shown="True" w685 {
          tunnel: w686 -> [w723 w736]
          tunnel: [w724 w727] -> w647
          tunnel: [w723 w728] -> w646
          tunnel: w687 -> [w724 w733]
          frame False {
          }
          frame True {
            w737 = u16 81  # Data Block #
            n193 = call "PADMINI_AUTO_BARCODE_STATUS 70.vi"("Enum"=enum16{"Read", "Write"}."Read", "error in (no error)"=w733) -> ("error out"=w732:errorcluster, "O/P"=w734:i32[])  [unwired: 8 in]
            n194 = global write "DATA LOG.vi" "OP 70 Outputs"(FALSE) -> ()
            n195 = call-poly <vilib>:"write DB.vi"("DINT input array"=w734, "error in (no error)"=w732, "Data Block #"=w737, "S7 Connection in"=w736) -> ("error out"=w725:errorcluster, "S7 Connection out"=w726:T4)  [unwired: 4 in, 2 out]
            n196 = call-poly <vilib>:"write DB.vi"("DINT input array"=i32[] [0] ("Data Byte"), "error in (no error)"=w725, "Data Block #"=u16 80, "S7 Connection in"=w726) -> ("error out"=w727:errorcluster, "S7 Connection out"=w728:T4)  [unwired: 4 in, 2 out]
          }
        }
        n197 = global read "DATA LOG.vi" "OP 70 reset"() -> (w648:bool)
        n198 = global read "DATA LOG.vi" "Auto Cycle On"() -> (w593:bool)
        n199 = case shown="True" w648 {
          tunnel: w647 -> [w698 w707]
          tunnel: [w698 w706] -> w637
          tunnel: w646 -> [w699 w705]
          tunnel: [w699 w704] -> w638
          frame False {
          }
          frame True {
            n200 = global write "DATA LOG.vi" "OP 70 reset"(FALSE) -> ()
            n201 = call-poly <vilib>:"write DB.vi"("Item offset [byte]"=u16 4 ("Data Block #"), "DINT input array"=i32[] [0], "error in (no error)"=w707, "Data Block #"=u16 80, "S7 Connection in"=w705) -> ("error out"=w706:errorcluster, "S7 Connection out"=w704:T4)  [unwired: 3 in, 2 out]
          }
        }
        n202 = Boolean To (0,1)(Boolean=w593) -> (0, 1=w592:i16)
        n203 = Build Array(w592) -> (w591:i16[])
        n204 = global read "Global 1.vi" "Filtered BARCODE selected"() -> (w639:string[])
        n205 = call-poly <vilib>:"write DB.vi"("Item offset [byte]"=u32 20, "DINT input array"=w591, "error in (no error)"=w637, "Data Block #"=w642, "S7 Connection in"=w638) -> ("error out"=w644:errorcluster, "S7 Connection out"=w645:T4)  [unwired: 3 in, 2 out]
        n206 = call-poly <vilib>:"write DB.vi"("Item offset [byte]"=u32 24, "Input STRINGS"=w639, "error in (no error)"=w644, "String length reserved in DB (default=254)"=u16 15, "Data Block #"=w642, "S7 Connection in"=w645) -> ("error out"=w635:errorcluster, "S7 Connection out"=w636:T4)  [unwired: 2 in, 2 out]
        n207 = call-poly <vilib>:"read DB.vi"("error in (no error)"=w635, "items #"=u16 2 ("Items # [byte]"), "Data Block #"=w623, "S7 Connection in"=w636) -> ("error out"=w683:errorcluster, "DINT result array"=w681:i32[], "S7 Connection out"=w678:T4)  [unwired: 5 in]
        n208 = call "PADMINI_AUTO_CYCLE STATE 70.vi"("Enum"=enum16{"Read", "Write"}."Write", "error in (no error)"=w683, "Input"=w681) -> ("error out"=w679:errorcluster)  [unwired: 7 in, 1 out]
        n209 = call-poly <vilib>:"read DB.vi"("Item offset [byte]"=u32 8, "error in (no error)"=w679, "items #"=u16 2 ("Items # [byte]"), "Data Block #"=w623, "S7 Connection in"=w678) -> ("error out"=w671:errorcluster, "REAL result array"=w669:sgl[], "S7 Connection out"=w677:T4)  [unwired: 4 in]
        n210 = call "PADMINI_AUTO_CYCLE VALUE 70.vi"("Enum"=enum16{"Read", "Write"}."Write", "error in (no error)"=w671, "Input"=w669) -> ("error out"=w670:errorcluster)  [unwired: 7 in, 1 out]
        n211 = call-poly <vilib>:"read DB.vi"("Item offset [byte]"=u32 16, "String length reserved in DB (default=254)"=u16 50, "error in (no error)"=w670, "items #"=u16 1 ("Items # [byte]"), "Data Block #"=w623, "S7 Connection in"=w677) -> ("error out"=w628:errorcluster, "STRING result Array"=w627:string[], "S7 Connection out"=w629:T4)  [unwired: 2 in, 1 out]
        n212 = call-poly <vilib>:"read DB.vi"("Item offset [byte]"=u32 68, "String length reserved in DB (default=254)"=u16 10, "error in (no error)"=w628, "items #"=u16 1 ("Items # [byte]"), "Data Block #"=w623, "S7 Connection in"=w629) -> ("error out"=w630:errorcluster, "STRING result Array"=w631:string[], "S7 Connection out"=w624:T4)  [unwired: 2 in, 1 out]
        n213 = Build Array (concatenate)(w627, w631) -> (w625:string[])
        n214 = call "PADMINI_AUTO_BARCODE_STRING 70.vi"("Enum"=enum16{"Read", "Write"}."Write", "error in (no error)"=w630, "Input"=w625) -> ("error out"=w650:errorcluster)  [unwired: 7 in, 1 out]
        n215 = global read "DATA LOG.vi" "OP 80 Outputs"() -> (w651:bool)
        n216 = case shown="True" w651 {
          tunnel: [w709 w712] -> w622
          tunnel: [w708 w713] -> w598
          tunnel: w650 -> [w709 w719]
          tunnel: w624 -> [w708 w716]
          frame False {
          }
          frame True {
            w722 = u16 83  # Data Block #
            n217 = call "PADMINI_AUTO_BARCODE_STATUS 80.vi"("Enum"=enum16{"Read", "Write"}."Read", "error in (no error)"=w719) -> ("error out"=w718:errorcluster, "O/P"=w720:i32[])  [unwired: 8 in]
            n218 = global write "DATA LOG.vi" "OP 80 Outputs"(FALSE) -> ()
            n219 = call-poly <vilib>:"write DB.vi"("DINT input array"=w720, "error in (no error)"=w718, "Data Block #"=w722, "S7 Connection in"=w716) -> ("error out"=w710:errorcluster, "S7 Connection out"=w711:T4)  [unwired: 4 in, 2 out]
            n220 = call-poly <vilib>:"write DB.vi"("DINT input array"=i32[] [0] ("Data Byte"), "error in (no error)"=w710, "Data Block #"=u16 82, "S7 Connection in"=w711) -> ("error out"=w712:errorcluster, "S7 Connection out"=w713:T4)  [unwired: 4 in, 2 out]
          }
        }
        n221 = global read "DATA LOG.vi" "OP 80 reset"() -> (w621:bool)
        n222 = global read "DATA LOG.vi" "Auto Cycle On"() -> (w596:bool)
        n223 = case shown="True" w621 {
          tunnel: w622 -> [w689 w697]
          tunnel: [w689 w692] -> _
          tunnel: [w689 w692] -> w611
          tunnel: w598 -> [w688 w691]
          tunnel: [w688 w690] -> w597
          frame False {
          }
          frame True {
            n224 = global write "DATA LOG.vi" "OP 80 reset"(FALSE) -> ()
            n225 = call-poly <vilib>:"write DB.vi"("Item offset [byte]"=u16 4 ("Data Block #"), "DINT input array"=i32[] [0], "error in (no error)"=w697, "Data Block #"=u16 82, "S7 Connection in"=w691) -> ("error out"=w692:errorcluster, "S7 Connection out"=w690:T4)  [unwired: 3 in, 2 out]
          }
        }
        n226 = Boolean To (0,1)(Boolean=w596) -> (0, 1=w595:i16)
        n227 = Build Array(w595) -> (w594:i16[])
        n228 = global read "Global 1.vi" "Filtered BARCODE selected"() -> (w614:string[])
        n229 = call-poly <vilib>:"write DB.vi"("Item offset [byte]"=u32 20, "DINT input array"=w594, "error in (no error)"=w611, "Data Block #"=w617, "S7 Connection in"=w597) -> ("error out"=w619:errorcluster, "S7 Connection out"=w620:T4)  [unwired: 3 in, 2 out]
        n230 = call-poly <vilib>:"write DB.vi"("Item offset [byte]"=u32 24, "Input STRINGS"=w614, "error in (no error)"=w619, "String length reserved in DB (default=254)"=u16 15, "Data Block #"=w617, "S7 Connection in"=w620) -> ("error out"=w612:errorcluster, "S7 Connection out"=w613:T4)  [unwired: 2 in, 2 out]
        n231 = call-poly <vilib>:"read DB.vi"("error in (no error)"=w612, "items #"=u16 2 ("Items # [byte]"), "Data Block #"=w600, "S7 Connection in"=w613) -> ("error out"=w653:errorcluster, "DINT result array"=w655:i32[], "S7 Connection out"=w658:T4)  [unwired: 5 in]
        n232 = call "PADMINI_AUTO_CYCLE STATE 80.vi"("Enum"=enum16{"Read", "Write"}."Write", "error in (no error)"=w653, "Input"=w655) -> ("error out"=w657:errorcluster)  [unwired: 7 in, 1 out]
        n233 = call-poly <vilib>:"read DB.vi"("Item offset [byte]"=u32 8, "error in (no error)"=w657, "items #"=u16 1 ("Items # [byte]"), "Data Block #"=w600, "S7 Connection in"=w658) -> ("error out"=w665:errorcluster, "REAL result array"=w667:sgl[], "S7 Connection out"=w659:T4)  [unwired: 4 in]
        n234 = call "PADMINI_AUTO_CYCLE VALUE 80.vi"("Enum"=enum16{"Read", "Write"}."Write", "error in (no error)"=w665, "Input"=w667) -> ("error out"=w666:errorcluster)  [unwired: 7 in, 1 out]
        n235 = call-poly <vilib>:"read DB.vi"("Item offset [byte]"=u32 12, "String length reserved in DB (default=254)"=u16 50, "error in (no error)"=w666, "items #"=u16 1 ("Items # [byte]"), "Data Block #"=w600, "S7 Connection in"=w659) -> ("error out"=w606:errorcluster, "STRING result Array"=w604:string[], "S7 Connection out"=w602:T4)  [unwired: 2 in, 1 out]
        n236 = call-poly <vilib>:"read DB.vi"("Item offset [byte]"=u32 64, "String length reserved in DB (default=254)"=u16 10, "error in (no error)"=w606, "items #"=u16 2 ("Items # [byte]"), "Data Block #"=w600, "S7 Connection in"=w602) -> ("error out"=w605:errorcluster, "STRING result Array"=w610:string[], "S7 Connection out"=w601:T4)  [unwired: 2 in, 1 out]
        n237 = Build Array (concatenate)(w604, w610) -> (w603:string[])
        n238 = call "PADMINI_AUTO_BARCODE_STRING 80.vi"("Enum"=enum16{"Read", "Write"}."Write", "error in (no error)"=w605, "Input"=w603) -> ("error out"=w649:errorcluster)  [unwired: 7 in, 1 out]
      }
      frame #1 {
        # "RECONNECT"
        n239 = case shown="Error" w741 {
          selector: w741 -> [w746 w754]
          tunnel: [w745 w751] -> w739
          tunnel: [w746 w752] -> w740
          tunnel: w742 -> [w745 w748]
          tunnel: w738 -> [_ w747]
          frame No Error {
          }
          frame Error {
            n240 = call <vilib>:"Clear Errors.vi"("error in (no error)"=w754) -> ("error out"=w755:errorcluster)  [unwired: 5 in, 1 out]
            n241 = call <vilib>:"disconnect.vi"("error in (no error)"=w755, "S7 Connection in"=w748) -> ("error out"=w753:errorcluster)  [unwired: 8 in, 1 out]
            n242 = call <vilib>:"Clear Errors.vi"("error in (no error)"=w753) -> ("error out"=w750:errorcluster)  [unwired: 5 in, 1 out]
            n243 = call <vilib>:"connect.vi"("PLC Type"=PLC_Type."S7 1200" ("PLC Type 2"), "error in (no error)"=w750, "IP address"=w747) -> ("error out"=w752:errorcluster, "S7 Connection out"=w751:T4)  [unwired: 7 in]
          }
        }
        n244 = Unbundle By Name(w741) -> ("status"=w744:bool)
        n245 = Not(x=w744) -> (.not. x?=w743:bool)
        "PLC 6" <- w743
        n246 = global write "Global 1.vi" "PLC 6"(w743) -> ()
      }
    }
    n247 = call "PADMINI_STOP_ALL.vi"("Enum"=enum16{"Read", "Write"}."Read") -> ("Boolean 2"=w584:bool)  [unwired: 9 in, 1 out]
    n248 = local read "stop"() -> (w583:bool)
    n249 = Or(x=w583, y=w584) -> (x .or. y?=w582:bool)
    n250 = Wait (ms)(milliseconds to wait=u32 50) -> ()  [unwired: 1 out]
  }
  n251 = while {
    shift-right: [w758] -> w72
    shift-left: w75 -> [w768]
    shift-right: [w766] -> w73
    shift-left: w76 -> [w767]
    tunnel: w71 -> [w757]
    stop <- w760 stop-if-true
    # "OP 60"
    n252 = flat-sequence {
      tunnel: [w777] -> w764
      tunnel: [w799] -> w759
      tunnel: w767 -> [w818]
      tunnel: w768 -> [w817]
      tunnel: w757 -> [w798]
      tunnel: [w798] -> w756
      tunnel: [w846] -> w766
      tunnel: [w845] -> w758
      tunnel: w764 -> [w848]
      tunnel: w759 -> [w847]
      tunnel: w756 -> [w844]
      frame #0 {
        w794 = u16 44 ("Data Block #")
        w774 = u16 43 ("Data Block #")
        # "AUTO WRITE"
        n253 = global read "DATA LOG.vi" "OP 60 Outputs"() -> (w816:bool)
        n254 = case shown="True" w816 {
          tunnel: w817 -> [w829 w842]
          tunnel: [w830 w831] -> w786
          tunnel: [w829 w834] -> w785
          tunnel: w818 -> [w830 w839]
          frame False {
          }
          frame True {
            w843 = u16 44  # Data Block #
            n255 = call "PADMINI_AUTO_BARCODE_STATUS 60.vi"("Enum"=enum16{"Read", "Write"}."Read", "error in (no error)"=w839) -> ("error out"=w838:errorcluster, "O/P"=w840:i32[])  [unwired: 8 in]
            n256 = global write "DATA LOG.vi" "OP 60 Outputs"(FALSE) -> ()
            n257 = call-poly <vilib>:"write DB.vi"("DINT input array"=w840, "error in (no error)"=w838, "Data Block #"=w843, "S7 Connection in"=w842) -> ("error out"=w832:errorcluster, "S7 Connection out"=w833:T4)  [unwired: 4 in, 2 out]
            n258 = call-poly <vilib>:"write DB.vi"("DINT input array"=i32[] [0] ("Data Byte"), "error in (no error)"=w832, "Data Block #"=u16 43, "S7 Connection in"=w833) -> ("error out"=w831:errorcluster, "S7 Connection out"=w834:T4)  [unwired: 4 in, 2 out]
          }
        }
        n259 = global read "DATA LOG.vi" "OP 60 reset"() -> (w784:bool)
        n260 = global read "DATA LOG.vi" "Auto Cycle On"() -> (w771:bool)
        n261 = case shown="True" w784 {
          tunnel: w786 -> [w819 w828]
          tunnel: [w819 w827] -> w787
          tunnel: w785 -> [w820 w826]
          tunnel: [w820 w825] -> w788
          frame False {
          }
          frame True {
            n262 = global write "DATA LOG.vi" "OP 60 reset"(FALSE) -> ()
            n263 = call-poly <vilib>:"write DB.vi"("Item offset [byte]"=u16 4 ("Data Block #"), "DINT input array"=i32[] [0], "error in (no error)"=w828, "Data Block #"=u16 43, "S7 Connection in"=w826) -> ("error out"=w827:errorcluster, "S7 Connection out"=w825:T4)  [unwired: 3 in, 2 out]
          }
        }
        n264 = Boolean To (0,1)(Boolean=w771) -> (0, 1=w770:i16)
        n265 = Build Array(w770) -> (w769:i16[])
        n266 = global read "Global 1.vi" "Filtered BARCODE selected"() -> (w797:string[])
        n267 = call-poly <vilib>:"write DB.vi"("Item offset [byte]"=u32 20, "DINT input array"=w769, "error in (no error)"=w787, "Data Block #"=w794, "S7 Connection in"=w788) -> ("error out"=w792:errorcluster, "S7 Connection out"=w791:T4)  [unwired: 3 in, 2 out]
        n268 = call-poly <vilib>:"write DB.vi"("Item offset [byte]"=u32 24, "Input STRINGS"=w797, "error in (no error)"=w792, "String length reserved in DB (default=254)"=u16 15, "Data Block #"=w794, "S7 Connection in"=w791) -> ("error out"=w789:errorcluster, "S7 Connection out"=w790:T4)  [unwired: 2 in, 2 out]
        n269 = call-poly <vilib>:"read DB.vi"("error in (no error)"=w789, "items #"=u16 2 ("Items # [byte]"), "Data Block #"=w774, "S7 Connection in"=w790) -> ("error out"=w814:errorcluster, "DINT result array"=w812:i32[], "S7 Connection out"=w809:T4)  [unwired: 5 in]
        n270 = call "PADMINI_AUTO_CYCLE STATE 60.vi"("Enum"=enum16{"Read", "Write"}."Write", "error in (no error)"=w814, "Input"=w812) -> ("error out"=w810:errorcluster)  [unwired: 7 in, 1 out]
        n271 = call-poly <vilib>:"read DB.vi"("Item offset [byte]"=u32 8, "error in (no error)"=w810, "items #"=u16 6 ("Items # [byte]"), "Data Block #"=w774, "S7 Connection in"=w809) -> ("error out"=w802:errorcluster, "REAL result array"=w800:sgl[], "S7 Connection out"=w808:T4)  [unwired: 4 in]
        n272 = call "PADMINI_AUTO_CYCLE VALUE 60.vi"("Enum"=enum16{"Read", "Write"}."Write", "error in (no error)"=w802, "Input"=w800) -> ("error out"=w801:errorcluster)  [unwired: 7 in, 1 out]
        n273 = call-poly <vilib>:"read DB.vi"("Item offset [byte]"=u32 32, "String length reserved in DB (default=254)"=u16 50, "error in (no error)"=w801, "items #"=u16 1 ("Items # [byte]"), "Data Block #"=w774, "S7 Connection in"=w808) -> ("error out"=w779:errorcluster, "STRING result Array"=w776:string[], "S7 Connection out"=w778:T4)  [unwired: 2 in, 1 out]
        n274 = call-poly <vilib>:"read DB.vi"("Item offset [byte]"=u32 84, "String length reserved in DB (default=254)"=u16 10, "error in (no error)"=w779, "items #"=u16 7 ("Items # [byte]"), "Data Block #"=w774, "S7 Connection in"=w778) -> ("error out"=w780:errorcluster, "STRING result Array"=w783:string[], "S7 Connection out"=w777:T4)  [unwired: 2 in, 1 out]
        n275 = Build Array (concatenate)(w776, w783) -> (w775:string[])
        n276 = call "PADMINI_AUTO_BARCODE_STRING 60.vi"("Enum"=enum16{"Read", "Write"}."Write", "error in (no error)"=w780, "Input"=w775) -> ("error out"=w799:errorcluster)  [unwired: 7 in, 1 out]
      }
      frame #1 {
        # "RECONNECT"
        n277 = case shown="Error" w847 {
          selector: w847 -> [w852 w860]
          tunnel: [w851 w857] -> w845
          tunnel: [w852 w858] -> w846
          tunnel: w848 -> [w851 w854]
          tunnel: w844 -> [_ w853]
          frame No Error {
          }
          frame Error {
            n278 = call <vilib>:"Clear Errors.vi"("error in (no error)"=w860) -> ("error out"=w861:errorcluster)  [unwired: 5 in, 1 out]
            n279 = call <vilib>:"disconnect.vi"("error in (no error)"=w861, "S7 Connection in"=w854) -> ("error out"=w859:errorcluster)  [unwired: 8 in, 1 out]
            n280 = call <vilib>:"Clear Errors.vi"("error in (no error)"=w859) -> ("error out"=w856:errorcluster)  [unwired: 5 in, 1 out]
            n281 = call <vilib>:"connect.vi"("PLC Type"=PLC_Type."S7 1200" ("PLC Type 2"), "error in (no error)"=w856, "IP address"=w853) -> ("error out"=w858:errorcluster, "S7 Connection out"=w857:T4)  [unwired: 7 in]
          }
        }
        n282 = Unbundle By Name(w847) -> ("status"=w850:bool)
        n283 = Not(x=w850) -> (.not. x?=w849:bool)
        "PLC 5" <- w849
        n284 = global write "Global 1.vi" "PLC 5"(w849) -> ()
      }
    }
    n285 = call "PADMINI_STOP_ALL.vi"("Enum"=enum16{"Read", "Write"}."Read") -> ("Boolean 2"=w762:bool)  [unwired: 9 in, 1 out]
    n286 = local read "stop"() -> (w761:bool)
    n287 = Or(x=w761, y=w762) -> (x .or. y?=w760:bool)
    n288 = Wait (ms)(milliseconds to wait=u32 50) -> ()  [unwired: 1 out]
  }
  n289 = while {
    shift-right: [w864] -> w110
    shift-left: w114 -> [w874]
    shift-right: [w872] -> w111
    shift-left: w115 -> [w873]
    tunnel: w113 -> [w863]
    stop <- w866 stop-if-true
    # "OP 40"
    n290 = flat-sequence {
      tunnel: [w886] -> w870
      tunnel: [w905] -> w865
      tunnel: w873 -> [w924]
      tunnel: w874 -> [w923]
      tunnel: w863 -> [w904]
      tunnel: [w904] -> w862
      tunnel: [w952] -> w872
      tunnel: [w951] -> w864
      tunnel: w870 -> [w954]
      tunnel: w865 -> [w953]
      tunnel: w862 -> [w950]
      frame #0 {
        w897 = u16 57 ("Data Block #")
        w885 = u16 56 ("Data Block #")
        # "AUTO WRITE"
        n291 = global read "DATA LOG.vi" "OP 40 Outputs"() -> (w922:bool)
        n292 = case shown="True" w922 {
          tunnel: w923 -> [w935 w948]
          tunnel: [w936 w940] -> w902
          tunnel: [w935 w942] -> w903
          tunnel: w924 -> [w936 w945]
          frame False {
          }
          frame True {
            w949 = u16 57  # Data Block #
            n293 = call "PADMINI_AUTO_BARCODE_STATUS 40.vi"("Enum"=enum16{"Read", "Write"}."Read", "error in (no error)"=w945) -> ("error out"=w944:errorcluster, "O/P"=w946:i32[])  [unwired: 8 in]
            n294 = global write "DATA LOG.vi" "OP 40 Outputs"(FALSE) -> ()
            n295 = call-poly <vilib>:"write DB.vi"("DINT input array"=w946, "error in (no error)"=w944, "Data Block #"=w949, "S7 Connection in"=w948) -> ("error out"=w939:errorcluster, "S7 Connection out"=w941:T4)  [unwired: 4 in, 2 out]
            n296 = call-poly <vilib>:"write DB.vi"("DINT input array"=i32[] [0], "error in (no error)"=w939, "Data Block #"=u16 56, "S7 Connection in"=w941) -> ("error out"=w940:errorcluster, "S7 Connection out"=w942:T4)  [unwired: 4 in, 2 out]
          }
        }
        n297 = global read "DATA LOG.vi" "OP 40 reset"() -> (w901:bool)
        n298 = global read "DATA LOG.vi" "Auto Cycle On"() -> (w877:bool)
        n299 = case shown="True" w901 {
          tunnel: w902 -> [w925 w934]
          tunnel: [w925 w933] -> w890
          tunnel: w903 -> [w926 w932]
          tunnel: [w926 w931] -> w891
          frame False {
          }
          frame True {
            n300 = global write "DATA LOG.vi" "OP 40 reset"(FALSE) -> ()
            n301 = call-poly <vilib>:"write DB.vi"("Item offset [byte]"=u16 4 ("Data Block #"), "DINT input array"=i32[] [0], "error in (no error)"=w934, "Data Block #"=u16 56, "S7 Connection in"=w932) -> ("error out"=w933:errorcluster, "S7 Connection out"=w931:T4)  [unwired: 3 in, 2 out]
          }
        }
        n302 = Boolean To (0,1)(Boolean=w877) -> (0, 1=w876:i16)
        n303 = Build Array(w876) -> (w875:i16[])
        n304 = global read "Global 1.vi" "Filtered BARCODE selected"() -> (w900:string[])
        n305 = call-poly <vilib>:"write DB.vi"("Item offset [byte]"=u32 20, "DINT input array"=w875, "error in (no error)"=w890, "Data Block #"=w897, "S7 Connection in"=w891) -> ("error out"=w895:errorcluster, "S7 Connection out"=w894:T4)  [unwired: 3 in, 2 out]
        n306 = call-poly <vilib>:"write DB.vi"("Item offset [byte]"=u32 24, "Input STRINGS"=w900, "error in (no error)"=w895, "String length reserved in DB (default=254)"=u16 15, "Data Block #"=w897, "S7 Connection in"=w894) -> ("error out"=w892:errorcluster, "S7 Connection out"=w893:T4)  [unwired: 2 in, 2 out]
        n307 = call-poly <vilib>:"read DB.vi"("error in (no error)"=w892, "items #"=u16 2 ("Items # [byte]"), "Data Block #"=w885, "S7 Connection in"=w893) -> ("error out"=w920:errorcluster, "DINT result array"=w918:i32[], "S7 Connection out"=w915:T4)  [unwired: 5 in]
        n308 = call "PADMINI_AUTO_CYCLE STATE 40.vi"("Enum"=enum16{"Read", "Write"}."Write", "error in (no error)"=w920, "Input"=w918) -> ("error out"=w916:errorcluster)  [unwired: 7 in, 1 out]
        n309 = call-poly <vilib>:"read DB.vi"("Item offset [byte]"=u32 8, "error in (no error)"=w916, "items #"=u16 4 ("Items # [byte]"), "Data Block #"=w885, "S7 Connection in"=w915) -> ("error out"=w908:errorcluster, "REAL result array"=w906:sgl[], "S7 Connection out"=w914:T4)  [unwired: 4 in]
        n310 = call "PADMINI_AUTO_CYCLE VALUE 40.vi"("Enum"=enum16{"Read", "Write"}."Write", "error in (no error)"=w908, "Input"=w906) -> ("error out"=w907:errorcluster)  [unwired: 7 in, 1 out]
        n311 = call-poly <vilib>:"read DB.vi"("Item offset [byte]"=u32 24, "String length reserved in DB (default=254)"=u16 50, "error in (no error)"=w907, "items #"=u16 1 ("Items # [byte]"), "Data Block #"=w885, "S7 Connection in"=w914) -> ("error out"=w889:errorcluster, "STRING result Array"=w880:string[], "S7 Connection out"=w887:T4)  [unwired: 2 in, 1 out]
        n312 = call-poly <vilib>:"read DB.vi"("Item offset [byte]"=u32 76, "String length reserved in DB (default=254)"=u16 10, "error in (no error)"=w889, "items #"=u16 4 ("Items # [byte]"), "Data Block #"=w885, "S7 Connection in"=w887) -> ("error out"=w888:errorcluster, "STRING result Array"=w879:string[], "S7 Connection out"=w886:T4)  [unwired: 2 in, 1 out]
        n313 = Build Array (concatenate)(w880, w879) -> (w878:string[])
        n314 = call "PADMINI_AUTO_BARCODE_STRING 40.vi"("Enum"=enum16{"Read", "Write"}."Write", "error in (no error)"=w888, "Input"=w878) -> ("error out"=w905:errorcluster)  [unwired: 7 in, 1 out]
      }
      frame #1 {
        # "RECONNECT"
        n315 = case shown="Error" w953 {
          selector: w953 -> [w958 w966]
          tunnel: [w957 w963] -> w951
          tunnel: [w958 w964] -> w952
          tunnel: w954 -> [w957 w960]
          tunnel: w950 -> [_ w959]
          frame No Error {
          }
          frame Error {
            n316 = call <vilib>:"Clear Errors.vi"("error in (no error)"=w966) -> ("error out"=w967:errorcluster)  [unwired: 5 in, 1 out]
            n317 = call <vilib>:"disconnect.vi"("error in (no error)"=w967, "S7 Connection in"=w960) -> ("error out"=w965:errorcluster)  [unwired: 8 in, 1 out]
            n318 = call <vilib>:"Clear Errors.vi"("error in (no error)"=w965) -> ("error out"=w962:errorcluster)  [unwired: 5 in, 1 out]
            n319 = call <vilib>:"connect.vi"("PLC Type"=PLC_Type."S7 1200" ("PLC Type 2"), "error in (no error)"=w962, "IP address"=w959) -> ("error out"=w964:errorcluster, "S7 Connection out"=w963:T4)  [unwired: 7 in]
          }
        }
        n320 = Unbundle By Name(w953) -> ("status"=w956:bool)
        n321 = Not(x=w956) -> (.not. x?=w955:bool)
        "PLC 3" <- w955
        n322 = global write "Global 1.vi" "PLC 3"(w955) -> ()
      }
    }
    n323 = call "PADMINI_STOP_ALL.vi"("Enum"=enum16{"Read", "Write"}."Read") -> ("Boolean 2"=w868:bool)  [unwired: 9 in, 1 out]
    n324 = local read "stop"() -> (w867:bool)
    n325 = Or(x=w867, y=w868) -> (x .or. y?=w866:bool)
    n326 = Wait (ms)(milliseconds to wait=u32 50) -> ()  [unwired: 1 out]
  }
  n327 = call <vilib>:"Clear Errors.vi"("error in (no error)"=w111) -> ("error out"=w112:errorcluster)  [unwired: 5 in, 1 out]
  n328 = call <vilib>:"Clear Errors.vi"("error in (no error)"=w120) -> ("error out"=w122:errorcluster)  [unwired: 5 in, 1 out]
  n329 = call <vilib>:"Clear Errors.vi"("error in (no error)"=w95) -> ("error out"=w94:errorcluster)  [unwired: 5 in, 1 out]
  n330 = call <vilib>:"Clear Errors.vi"("error in (no error)"=w73) -> ("error out"=w74:errorcluster)  [unwired: 5 in, 1 out]
  n331 = call <vilib>:"disconnect.vi"("error in (no error)"=w112, "S7 Connection in"=w110) -> ("error out"=w109:errorcluster)  [unwired: 8 in, 1 out]
  n332 = call <vilib>:"disconnect.vi"("error in (no error)"=w122, "S7 Connection in"=w121) -> ("error out"=w108:errorcluster)  [unwired: 8 in, 1 out]
  n333 = call <vilib>:"disconnect.vi"("error in (no error)"=w94, "S7 Connection in"=w96) -> ("error out"=w70:errorcluster)  [unwired: 8 in, 1 out]
  n334 = call <vilib>:"disconnect.vi"("error in (no error)"=w74, "S7 Connection in"=w72) -> ("error out"=w69:errorcluster)  [unwired: 8 in, 1 out]
  n335 = Merge Errors(w108, w109, w70, w69) -> (w107:errorcluster)
  n336 = call <vilib>:"Clear Errors.vi"("error in (no error)"=w53) -> ("error out"=w54:errorcluster)  [unwired: 5 in, 1 out]
  n337 = call <vilib>:"disconnect.vi"("error in (no error)"=w54, "S7 Connection in"=w52) -> ("error out"=w22:errorcluster)  [unwired: 8 in, 1 out]
  n338 = call <vilib>:"Clear Errors.vi"("error in (no error)"=w163) -> ("error out"=w149:errorcluster)  [unwired: 5 in, 1 out]
  n339 = call <vilib>:"disconnect.vi"("error in (no error)"=w149, "S7 Connection in"=w148) -> ("error out"=w147:errorcluster)  [unwired: 8 in, 1 out]
  n340 = control-ref of="This VI"() -> (w3:refnum<vi>)
  n341 = call <vilib>:"Clear Errors.vi"("error in (no error)"=w24) -> ("error out"=w25:errorcluster)  [unwired: 5 in, 1 out]
  n342 = call <vilib>:"disconnect.vi"("error in (no error)"=w25, "S7 Connection in"=w23) -> ("error out"=w20:errorcluster)  [unwired: 8 in, 1 out]
  n343 = Merge Errors(w22, w20) -> (w21:errorcluster)
  n344 = Merge Errors(w147, w107, w21) -> (w168:errorcluster)
  n345 = call <vilib>:"Simple Error Handler.vi"("type of dialog (OK msg:1)"=w2, "error in (no error)"=w168) -> ("error out"=w167:errorcluster)  [unwired: 3 in, 4 out]
  n346 = call <vilib>:"Clear Errors.vi"("error in (no error)"=w167) -> ("error out"=w166:errorcluster)  [unwired: 5 in, 1 out]
  n347 = invoke class="VI" method="FP.Close"(reference=w3, error in=w166) -> (error out=→"error out":errorcluster)  [unwired: 1 in, 2 out]
